vi "LD2018_ブロック崩し_ステージセット.vi"(9 "Stage":i32, 10 "Position":T1, 11 "ブロックReference":refnum<vi>[][](array[refnum])) -> (2 "ブッロク配列":bool[][](array[boolean]), 3 "ブロックReference":refnum<vi>[][](array[refnum]))   [LabVIEW 2016]
uses:
  <vilib>/Utility/miscctls.llb/LVPositionTypeDef.ctl
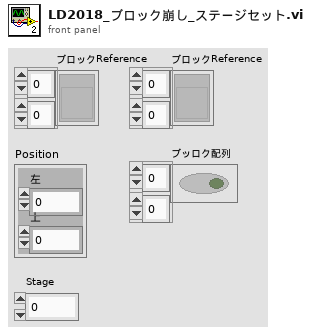
[diagram p1: front panel]
types:
  T1 = typedef "LVPositionTypeDef.ctl" = cluster{"Left":i32, "Top":i32}
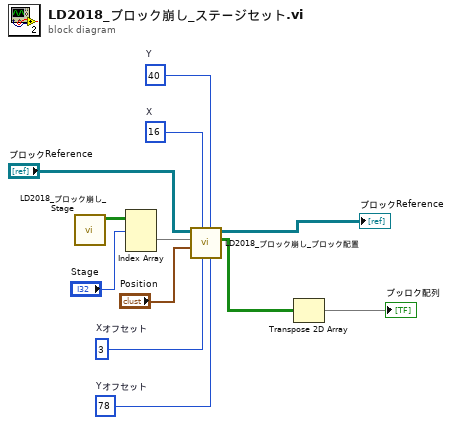
[diagram p0: block diagram]
diagram:
  w7 = 78  # Yオフセット
  w6 = 3  # Xオフセット
  w5 = 40  # Y
  w4 = 16  # X
  n1 = call "LD2018_ブロック崩し_Stage.vi"() -> ("Stages"=w10:bool[][][])  [unwired: 11 in]
  n2 = Index Array(array=w10, index (dim 0)="Stage") -> (element=w12:bool[][])  [unwired: 2 in]
  n3 = call "LD2018_ブロック崩し_ブロック配置.vi"("Yオフセット"=w7, "Y"=w5, "Xオフセット"=w6, "X"=w4, "Scrn-BALL位置"="Position", "ブロック配列入力"=w12, "ブッロクReference"="ブロックReference") -> ("ブロック配列出力"=w9:bool[][], "ブッロクReference出力"=→"ブロックReference":refnum<vi>[][])  [unwired: 3 in]
  n4 = Transpose 2D Array(2D array=w9) -> (transposed array=→"ブッロク配列":bool[][])
